vi "Advanced VI Tree - Caraya.vi"   [LabVIEW 2013]
doc: "Advanced VI Tree of the public supported methods of Caraya Unit Test Framework"
uses:
  classes/Test Runner/Test Runner.lvclass
  tests/test-TestableClass/Caraya-TestableClass.lvclass
  classes/Test Runner/Test Runner.lvclass/Test Runner.ctl
  classes/Test Suite/Test Suite.lvclass
  run-tests/Run Test (Scalar Path).vi
  run-tests/Run Test (Array Path).vi
  run-tests/Run Test (VIRefnum Scalar).vi
  run-tests/Run Test (VIRefnum Array).vi
  run-tests/Run Test (ProjectRefnum).vi
  run-tests/Run Test (Object Array).vi
  run-tests/Run Test (Object).vi
  run-tests/Run Test (LibraryRefnum).vi
  classes/Test Suite/Define Test Suite (Default).vi
  classes/Assert/Assert.lvclass
  classes/Basic Test Manager/Basic Test Manager.lvclass
  classes/Test Runner.Collection/Test Runner.Collection.lvclass
  classes/Test Runner.Project/Test Runner.Project.lvclass
  classes/Test Runner.Folder/Test Runner.Folder.lvclass
  tests/test-runner/test-all-asserts/Test Runner.AllAsserts.lvclass
  tests/test-runner/UnitTest For Runner/Unit Tests for Runner.lvclass
  Caraya.lvlib
  classes/Test Report.Default/Test Report.Default.lvclass
  classes/Test Report.JUnit/Test Report.JUnit.lvclass
  classes/Test/Test.lvclass
  classes/Test Runner.Class/Test Runner.Class.lvclass
  classes/Test Result/Test Result.lvclass
  classes/Properties/Properties.lvclass
types:
  T1 = typedef "Caraya.lvlib/Test Result.lvclass/Assert Event Data.ctl" = cluster{"Name":string, "Passed":bool, "Call Chain":string[], "Test Error":errorcluster, "Time Stamp":timestamp, "Unique Assert ID":string, "Test ID":string, "Execution time (s)":dbl, "Verbose Explanation":string, "properties":variant, "measurements":variant, "limits":variant}
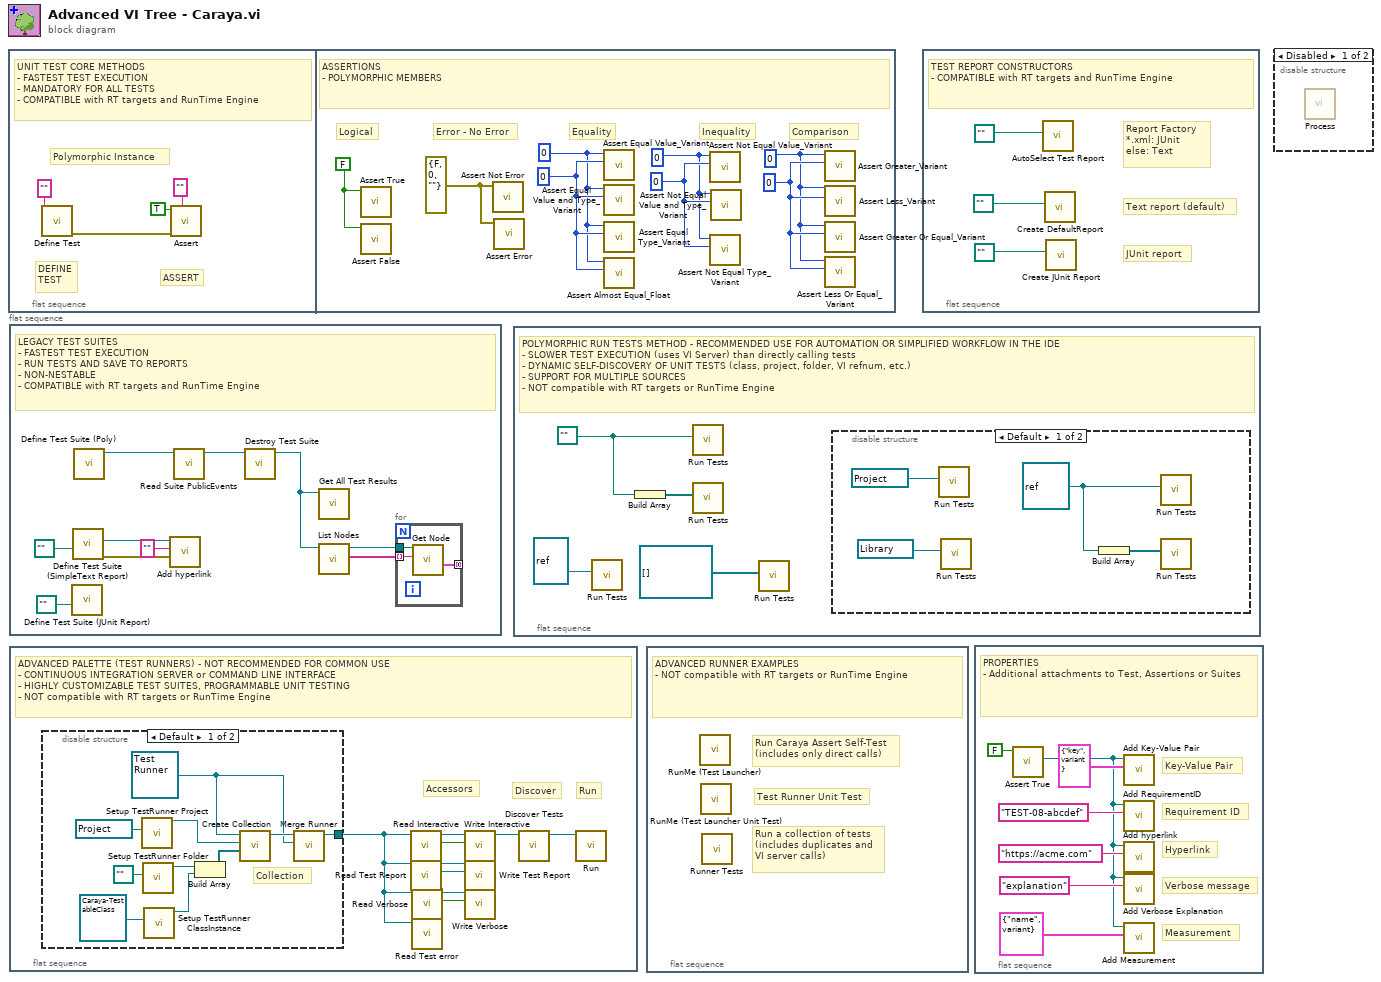
[diagram p0: block diagram]
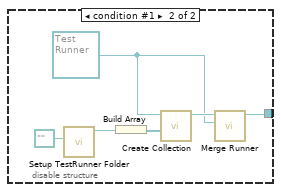
[diagram p3: hidden frame]
diagram:
  n1 = flat-sequence {
    frame #0 {
      # "ASSERT"
      # "DEFINE\nTEST"
      # "Polymorphic Instance"
      # "UNIT TEST CORE METHODS\n- FASTEST TEST EXECUTION\n- MANDATORY FOR ALL TESTS\n- COMPATIBLE with RT targets and RunTime Engine"
      n2 = call "Define Test.vi"("Label (VI Title)"="") -> ("error out"=w1:errorcluster)  [unwired: 9 in, 1 out]
      n3 = call-poly "Assert.vi"("Label"="" ("Label (VI Title)"), "error in (no error)"=w1, "True?"=TRUE) -> ()  [unwired: 7 in, 2 out]
    }
    frame #1 {
      w6 = errorcluster {"status"=FALSE, "code"=0, "source"=""} ("Error?")
      w5 = FALSE ("True?")
      w8 = 0
      w7 = 0
      w10 = 0
      w9 = 0
      w12 = 0
      w11 = 0
      # "Error - No Error"
      # "Logical"
      # "Equality"
      # "Inequality"
      # "Comparison"
      # "ASSERTIONS\n- POLYMORPHIC MEMBERS"
      n4 = call "Assert True.vi"("True?"=w5) -> ()  [unwired: 9 in, 2 out]
      n5 = call "Assert False.vi"("False?"=w5) -> ()  [unwired: 9 in, 2 out]
      n6 = call "Assert Not Error.vi"("Not Error?"=w6) -> ()  [unwired: 9 in, 2 out]
      n7 = call "Assert Error.vi"("Error?"=w6) -> ()  [unwired: 9 in, 2 out]
      n8 = call "Assert Equal Value_Variant.vi"("Y"=w8, "X"=w7) -> ()  [unwired: 8 in, 2 out]
      n9 = call "Assert Equal Value and Type_Variant.vi"("Y"=w8, "X"=w7) -> ()  [unwired: 8 in, 2 out]
      n10 = call "Assert Equal Type_Variant.vi"("Y"=w8, "X"=w7) -> ()  [unwired: 8 in, 2 out]
      n11 = call "Assert Almost Equal_Float.vi"("Y"=w8, "X"=w7) -> ()  [unwired: 8 in, 2 out]
      n12 = call "Assert Not Equal Value_Variant.vi"("Y"=w10, "X"=w9) -> ()  [unwired: 8 in, 2 out]
      n13 = call "Assert Not Equal Type_Variant.vi"("Y"=w10, "X"=w9) -> ()  [unwired: 8 in, 2 out]
      n14 = call "Assert Not Equal Value and Type_Variant.vi"("Y"=w10, "X"=w9) -> ()  [unwired: 8 in, 2 out]
      n15 = call "Assert Greater_Variant.vi"("Y"=w12, "X"=w11) -> ()  [unwired: 8 in, 2 out]
      n16 = call "Assert Less_Variant.vi"("Y"=w12, "X"=w11) -> ()  [unwired: 8 in, 2 out]
      n17 = call "Assert Greater Or Equal_Variant.vi"("Y"=w12, "X"=w11) -> ()  [unwired: 8 in, 2 out]
      n18 = call "Assert Less Or Equal_Variant.vi"("Y"=w12, "X"=w11) -> ()  [unwired: 8 in, 2 out]
    }
  }
  n19 = flat-sequence {
    frame #0 {
      # "LEGACY TEST SUITES\n- FASTEST TEST EXECUTION\n- RUN TESTS AND SAVE TO REPORTS\n- NON-NESTABLE\n- COMPATIBLE with RT targets and RunTime Engine"
      n20 = call "Define Test Suite (JUnit Report).vi"("Report Path"=path "") -> ()  [unwired: 8 in, 3 out]
      n21 = call "Define Test Suite (SimpleText Report).vi"("Report Path"=path "") -> ("error out"=w14:errorcluster, "Properties.Suite"=w15:refnum<class "Properties.Suite.lvclass">)  [unwired: 8 in, 1 out]
      n22 = call-poly "Define Test Suite (Poly).vi"() -> ("Test Suite"=w20:refnum<class "Test Suite.lvclass">)  [unwired: 9 in, 2 out]
      n23 = call "Add hyperlink.vi"("error in (no error)"=w14, "URL"="", "Properties"=w15) -> ()  [unwired: 7 in, 2 out]
      n24 = call "Read Suite PublicEvents.vi"("Test Suite in"=w20) -> ("Test Suite out"=w19:refnum<class "Test Suite.lvclass">)  [unwired: 8 in, 2 out]
      n25 = call-dynamic "Destroy Test Suite.vi"("Test Suite in"=w19) -> ("Test Suite Results"=w18:refnum<class "Test Result.lvclass">)  [unwired: 9 in, 1 out]
      n26 = call "Get All Test Results.vi"("Test Result in"=w18) -> ()  [unwired: 8 in, 3 out]
      n27 = call "List Nodes.vi"("Test Result in"=w18) -> ("Nodes"=w16:string[], "Test Result out"=w17:refnum<class "Test Result.lvclass">)  [unwired: 8 in, 1 out]
      n28 = for {
        tunnel: w17 -> [w25]
        tunnel: w16 -> [w24] mode=indexing
        tunnel: [w23] -> _ mode=concatenating
        n29 = call "Get Node.vi"("Node"=w24, "Test Result in"=w25) -> ("Assertions"=w23:T1[])  [unwired: 4 in, 5 out]
      }
    }
  }
  n30 = flat-sequence {
    frame #0 {
      # "Run"
      # "Discover"
      # "Accessors"
      # "ADVANCED PALETTE (TEST RUNNERS) - NOT RECOMMENDED FOR COMMON USE\n- CONTINUOUS INTEGRATION SERVER or COMMAND LINE INTERFACE\n- HIGHLY CUSTOMIZABLE TEST SUITES, PROGRAMMABLE UNIT TESTING\n- NOT compatible with RT targets or RunTime Engine"
      n31 = disable-structure shown="Default" {
        disable-tunnel: [w37 w45] -> w34
        frame condition #0 (active) {
          w38 = refnum<class "Test Runner.lvclass"> refnum ("Caraya.lvlib:Test Runner.lvclass")
          # "Collection"
          n32 = call "Setup TestRunner Project.vi"("Project Refnum"=refnum<vi> refnum) -> ("Test Runner.Project out"=w42:refnum<class "Test Runner.Project.lvclass">)  [unwired: 9 in, 1 out]
          n33 = call "Setup TestRunner Folder.vi"("Directory to search"=path "") -> ("Test Runner.Folder out"=w41:refnum<class "Test Runner.Folder.lvclass">)  [unwired: 9 in, 1 out]
          n34 = call "Setup TestRunner ClassInstance.vi"("Instance"=refnum<class "Caraya-TestableClass.lvclass"> refnum ("Caraya-TestableClass.lvclass")) -> ("Test Runner.Class out"=w35:refnum<class "Test Runner.Class.lvclass">)  [unwired: 9 in, 1 out]
          n35 = Build Array(w41, w35) -> (w40:refnum<class "Test Runner.lvclass">[])
          n36 = call "Create Collection.vi"("Test Runners"=w40, "Test Runner 2"=w42, "Test Runner 1"=w38) -> ("Test Runner.Collection out"=w39:refnum<class "Test Runner.Collection.lvclass">)  [unwired: 7 in, 1 out]
          n37 = call "Merge Runner.vi"("Test Runner"=w38, "Test Runner.Collection in"=w39) -> ("Test Runner.Collection out"=w37:refnum<class "Test Runner.Collection.lvclass">)  [unwired: 9 in]
        }
        frame condition #1 {
          w46 = refnum<class "Test Runner.lvclass"> refnum ("Caraya.lvlib:Test Runner.lvclass")
          n38 = call "Setup TestRunner Folder.vi"("Directory to search"=path "") -> ("Test Runner.Folder out"=w49:refnum<class "Test Runner.Folder.lvclass">)  [unwired: 9 in, 1 out]
          n39 = Build Array(w49) -> (w48:refnum<class "Test Runner.Folder.lvclass">[])
          n40 = call "Create Collection.vi"("Test Runners"=w48, "Test Runner 1"=w46) -> ("Test Runner.Collection out"=w47:refnum<class "Test Runner.Collection.lvclass">)  [unwired: 8 in, 1 out]
          n41 = call "Merge Runner.vi"("Test Runner"=w46, "Test Runner.Collection in"=w47) -> ("Test Runner.Collection out"=w45:refnum<class "Test Runner.Collection.lvclass">)  [unwired: 9 in]
        }
      }
      n42 = call "Read Interactive.vi"("Test Runner in"=w34) -> ("Interactive"=w30:bool, "Test Runner out"=w29:refnum<class "Test Runner.Collection.lvclass">)  [unwired: 9 in]
      n43 = call "Read Test Report.vi"("Test Runner in"=w34) -> ("Test Report"=w32:refnum<class "Test Report.lvclass">, "Test Runner out"=w31:refnum<class "Test Runner.Collection.lvclass">)  [unwired: 8 in, 1 out]
      n44 = call "Read Verbose.vi"("Test Runner in"=w34) -> ("Verbose"=w28:bool, "Test Runner out"=w27:refnum<class "Test Runner.Collection.lvclass">)  [unwired: 9 in]
      n45 = call "Read Test error.vi"("Test Runner in"=w34) -> ()  [unwired: 8 in, 3 out]
      n46 = call "Write Interactive.vi"("Interactive"=w30, "Test Runner in"=w29) -> ("Test Runner out"=w33:refnum<class "Test Runner.Collection.lvclass">)  [unwired: 9 in]
      n47 = call "Write Test Report.vi"("Test Report"=w32, "Test Runner in"=w31) -> ()  [unwired: 9 in, 1 out]
      n48 = call "Write Verbose.vi"("Verbose"=w28, "Test Runner in"=w27) -> ()  [unwired: 9 in, 1 out]
      n49 = call "Discover Tests.vi"("Test Runner in"=w33) -> ("Test Runner out"=w26:refnum<class "Test Runner.Collection.lvclass">)  [unwired: 9 in, 1 out]
      n50 = call "Run.vi"("Test Runner in"=w26) -> ()  [unwired: 8 in, 3 out]
    }
  }
  n51 = flat-sequence {
    frame #0 {
      w53 = path "" ("Test Path")
      # "POLYMORPHIC RUN TESTS METHOD - RECOMMENDED USE FOR AUTOMATION OR SIMPLIFIED WORKFLOW IN THE IDE\n- SLOWER TEST EXECUTION (uses VI Server) than directly calling tests\n- DYNAMIC SELF-DISCOVERY OF UNIT TESTS (class, project, folder, VI refnum, etc.)\n- SUPPORT FOR MULTIPLE SOURCES\n- NOT compatible with RT targets or RunTime Engine"
      n52 = call-poly "Run Tests.vi"("VI Refnum"=refnum<vi> refnum) -> ()  [unwired: 9 in, 2 out]
      n53 = Build Array(w53) -> (w54:path[])
      n54 = call-poly "Run Tests.vi"("Test Path"=w53) -> ()  [unwired: 9 in, 2 out]
      n55 = call-poly "Run Tests.vi"("Paths"=w54) -> ()  [unwired: 9 in, 2 out]
      n56 = call-poly "Run Tests.vi"("VI Refnums"=refnum<vi>[] []) -> ()  [unwired: 9 in, 2 out]
      n57 = disable-structure shown="Default" {
        frame condition #0 (active) {
          w56 = refnum<class> refnum ("Object")
          n58 = call-poly "Run Tests.vi"("Project Refnum"=refnum<vi> refnum) -> ()  [unwired: 9 in, 2 out]
          n59 = call-poly "Run Tests.vi"("Library Refnum"=refnum<vi> refnum) -> ()  [unwired: 9 in, 2 out]
          n60 = Build Array(w56) -> (w57:refnum<class>[])
          n61 = call-poly "Run Tests.vi"("Object"=w56) -> ()  [unwired: 9 in, 2 out]
          n62 = call-poly "Run Tests.vi"("Objects"=w57) -> ()  [unwired: 9 in, 2 out]
        }
        frame condition #1 {
        }
      }
    }
  }
  n63 = flat-sequence {
    frame #0 {
      # "Run a collection of tests\n(includes duplicates and\nVI server calls)"
      # "Test Runner Unit Test"
      # "Run Caraya Assert Self-Test\n(includes only direct calls)"
      # "ADVANCED RUNNER EXAMPLES\n- NOT compatible with RT targets or RunTime Engine"
      n64 = call "RunMe (Test Launcher).vi"() -> ()  [unwired: 12 in]
      n65 = call "RunMe (Test Launcher Unit Test).vi"() -> ()  [unwired: 12 in]
      n66 = call "Runner Tests.vi"() -> ()  [unwired: 11 in, 1 out]
    }
  }
  n67 = flat-sequence {
    frame #0 {
      # "Report Factory\n*.xml: JUnit\nelse: Text"
      # "JUnit report"
      # "Text report (default)"
      # "TEST REPORT CONSTRUCTORS\n- COMPATIBLE with RT targets and RunTime Engine"
      n68 = call "AutoSelect Test Report.vi"("Report Path"=path "") -> ()  [unwired: 9 in, 2 out]
      n69 = call "Create DefaultReport.vi"("Report Path"=path "") -> ()  [unwired: 9 in, 2 out]
      n70 = call "Create JUnit Report.vi"("Report Path"=path "") -> ()  [unwired: 9 in, 2 out]
    }
  }
  n71 = flat-sequence {
    frame #0 {
      # "Measurement"
      # "Verbose message"
      # "Hyperlink"
      # "Requirement ID"
      # "Key-Value Pair"
      # "PROPERTIES\n- Additional attachments to Test, Assertions or Suites"
      n72 = call "Assert True.vi"("True?"=FALSE) -> ("Properties"=w62:refnum<class "Properties.Assert.lvclass">)  [unwired: 9 in, 1 out]
      n73 = call "Add Key-Value Pair.vi"("entry"=cluster{"key":string, "value":variant} {"key"="key", "value"=variant}, "Properties in"=w62) -> ()  [unwired: 8 in, 2 out]
      n74 = call "Add RequirementID.vi"("Requirement ID"="TEST-08-abcdef", "Properties"=w62) -> ()  [unwired: 8 in, 2 out]
      n75 = call "Add hyperlink.vi"("URL"="https://acme.com", "Properties"=w62) -> ()  [unwired: 8 in, 2 out]
      n76 = call "Add Verbose Explanation.vi"("Verbose Explanation"="explanation", "Properties"=w62) -> ()  [unwired: 8 in, 2 out]
      n77 = call "Add Measurement.vi"("entry"=cluster{"key":string, "value":variant} {"key"="name", "value"=variant}, "Properties"=w62) -> ()  [unwired: 8 in, 2 out]
    }
  }
  n78 = disable-structure shown="Disabled" {
    frame Disabled {
      n79 = call "Process.vi"() -> ()  [unwired: 10 in, 2 out]
    }
    frame Enabled {
    }
  }
